vi "MIDAS_ODB_Add_Or_Update.vi"(8 "Input Array":T1[](array[typedef]), 11 "input cluster":T1) -> (0 "Output Array":T1[](array[typedef]), 3 "Entry Already Exists":bool)   [LabVIEW 2018, in "feGEM DataPacker.lvlib"]
uses:
  MIDAS_ODB_Entry.ctl
  feGEM DataPacker.lvlib
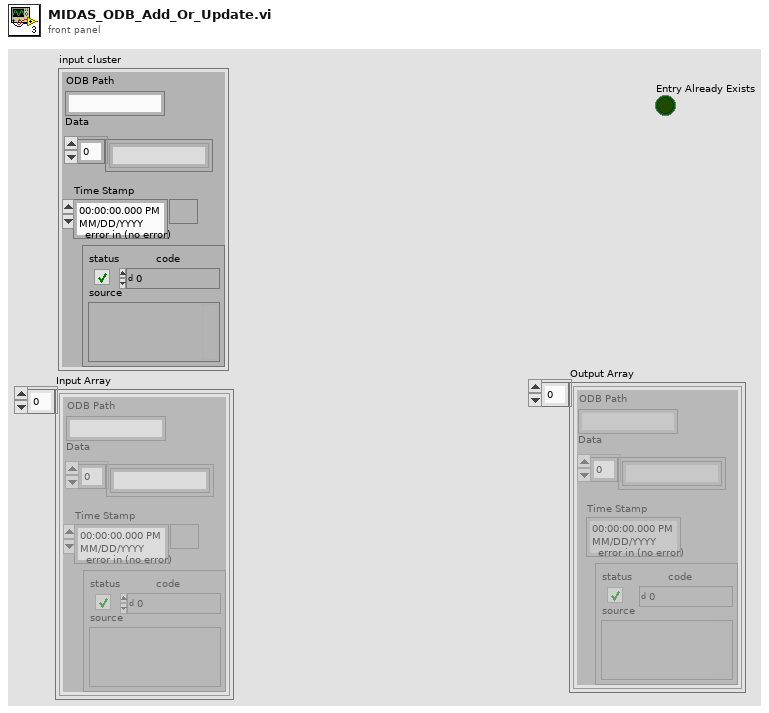
[diagram p1: front panel]
types:
  T1 = typedef "feGEM DataPacker.lvlib/MIDAS_ODB_Entry.ctl" = cluster{"ODB Path":string, "Data":string[], "Time Stamp":timestamp, "error in (no error)":errorcluster}
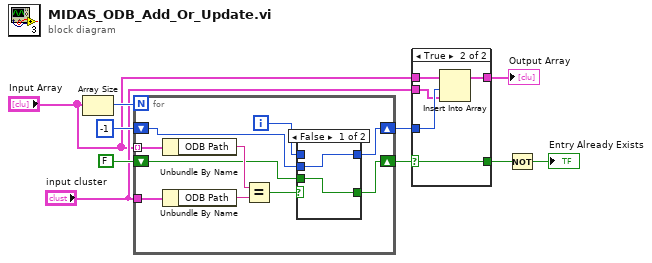
[diagram p0: block diagram]
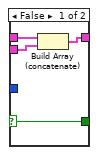
[diagram p2: hidden frame]
diagram:
  n1 = Array Size(array="Input Array") -> (size(s)=w10:i32)
  n2 = for {
    N: w10 -> [_]
    tunnel: "Input Array" -> [w20] mode=indexing
    tunnel: "input cluster" -> [w18]
    shift-right: [w14] -> w6
    shift-left: -1 -> [w13]
    shift-right: [w12] -> w7
    shift-left: FALSE -> [w11]
    i -> [w15]
    n3 = Unbundle By Name(w20) -> ("ODB Path"=w19:string)
    n4 = Unbundle By Name(w18) -> ("ODB Path"=w17:string)
    n5 = Equal?(x=w19, y=w17) -> (x = y?=w16:bool)
    n6 = case shown="False" w16 {
      selector: w16 -> [_ w23]
      tunnel: w15 -> [_ w24]
      tunnel: [w22 w24] -> w14
      tunnel: w13 -> [w22 _]
      tunnel: [w21 w23] -> w12
      tunnel: w11 -> [w21 _]
      frame False {
      }
      frame True {
      }
    }
  }
  n7 = case shown="True" w7 {
    selector: w7 -> [w25 w29]
    tunnel: w6 -> [_ w33]
    tunnel: "input cluster" -> [w27 w32]
    tunnel: "Input Array" -> [w28 w31]
    tunnel: [w26 w30] -> w3
    tunnel: [w25 w29] -> w2
    frame False {
      n8 = Build Array (concatenate)(w28, w27) -> (w26:T1[])
    }
    frame True {
      n9 = Insert Into Array(array=w31, index=w33, new element=w32) -> (w30:T1[])
    }
  }
  "Output Array" <- w3
  n10 = Not(x=w2) -> (.not. x?=→"Entry Already Exists":bool)
